vi "Apend Error Result to Case Element.vi"(8 "error in (no error)":errorcluster, 9 "Method Result":T1, 10 "Test Case Element in":refnum<k20>, 11 "XML Report In":refnum<class "XML Report.lvclass">) -> (0 "error out":errorcluster, 2 "Test Case Element out":refnum<k20>, 3 "XML Report Out":refnum<class "XML Report.lvclass">)   [LabVIEW 2020, in "XML Report.lvclass"]
uses:
  XML Report.lvclass
  <resource>/objmgr/DOMUserDefRef.rc
  <vilib>/xml/NI_XML.lvlib
  <vilib>/xml/Close Reference(Node).vi
  Result Types/Assertion Result/Public/TypeDefs/Status.ctl
  Result Types/Assertion Result/Assertion Result.lvlib
  Result Types/Assertion Result/Public/TypeDefs/Assertion Type.ctl
  Result Types/Assertion Result/Assertion Result.ctl
  Result Types/Method Result/Method Result.ctl
  Result Types/Method Result/Method Result.lvlib
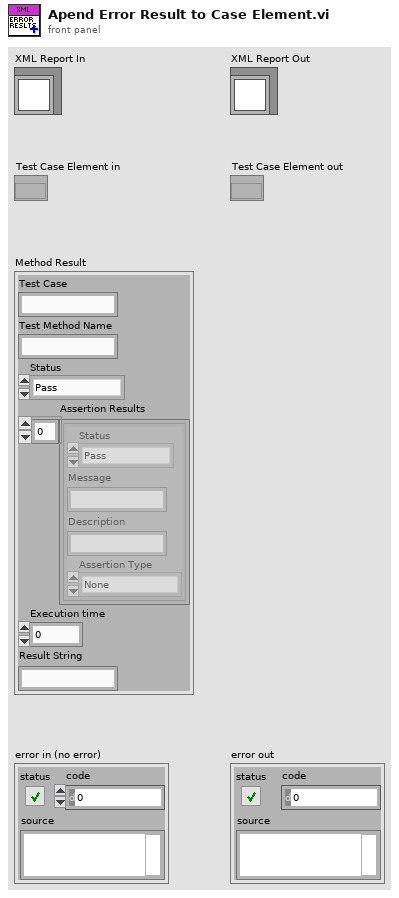
[diagram p1: front panel]
types:
  T1 = typedef "Method Result.lvlib/Method Result.ctl" = cluster{"Test Case":string, "Test Method Name":string, "Status":T2, "Assertion Results":T3[], "Execution time":dbl, "Result String":string}
  T2 = typedef "Assertion Result.lvlib/Status.ctl" = enum16{"Pass", "Fail", "Error", "Skipped", "Setup Error", "Broken", "Teardown Error"}
  T3 = typedef "Assertion Result.lvlib/Assertion Result.ctl" = cluster{"Status":T2, "Message":string, "Description":string, "Assertion Type":T4}
  T4 = typedef "Assertion Result.lvlib/Assertion Type.ctl" = enum16{"None", "Pass", "Fail", "Skip", "Pass if Equal", "Fail if Equal", "Pass if Error", "Fail if Error", "Pass if", "Fail if"}
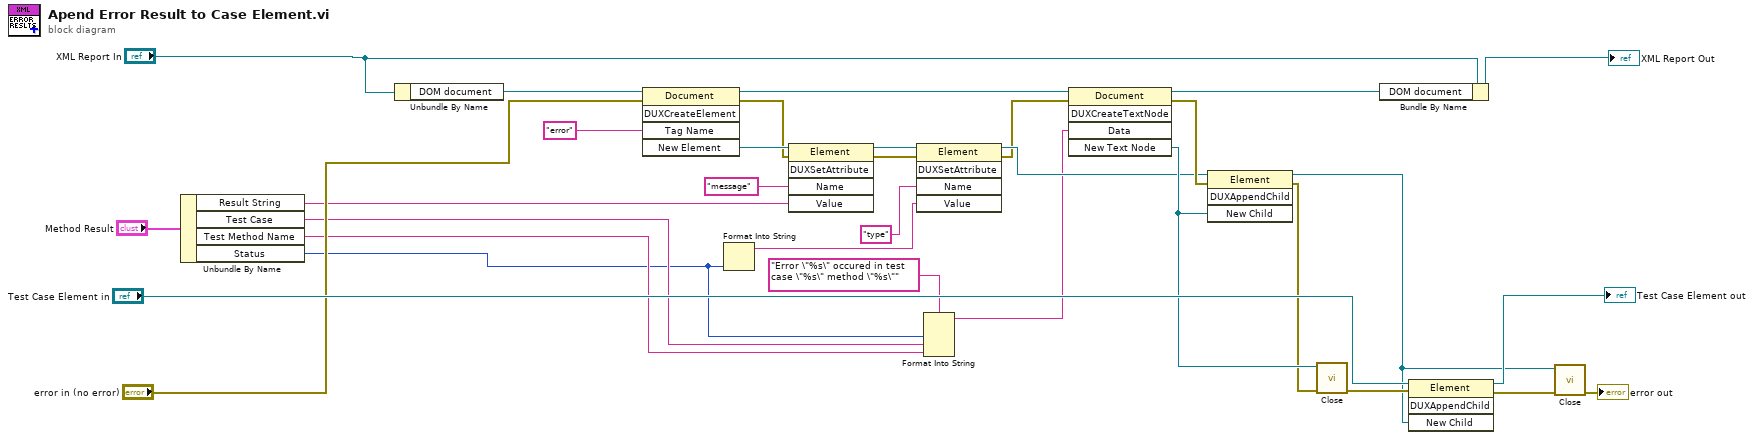
[diagram p0: block diagram]
diagram:
  n1 = Unbundle By Name("Method Result") -> ("Result String"=w5:string, "Test Case"=w3:string, "Test Method Name"=w2:string, "Status"=w1:T2)
  n2 = Unbundle By Name("XML Report In") -> ("DOM document"=w27:refnum<k20>)
  n3 = invoke class="Document" method="DUXCreateElement"(reference=w27, error in="error in (no error)", "Tag Name"="error") -> (reference out=w20:refnum<k20>, error out=w24:errorcluster, "New Element"=w25:refnum<k20>)  [unwired: 2 in, 2 out]
  n4 = Format Into String(w1) -> (resulting string=w9:string)  [unwired: 3 in, 1 out]
  n5 = invoke class="Element" method="DUXSetAttribute"(reference=w25, error in=w24, "Name"="message", "Value"=w5) -> (reference out=w13:refnum<k20>, error out=w11:errorcluster)  [unwired: 1 in, 3 out]
  n6 = invoke class="Element" method="DUXSetAttribute"(reference=w13, error in=w11, "Name"="type", "Value"=w9) -> (reference out=w12:refnum<k20>, error out=w10:errorcluster)  [unwired: 1 in, 3 out]
  n7 = Format Into String(format string="Error \"%s\" occured in test case \"%s\" method \"%s\"", w1, w3, w2) -> (resulting string=w7:string)  [unwired: 2 in, 1 out]
  n8 = invoke class="Document" method="DUXCreateTextNode"(reference=w20, error in=w10, "Data"=w7) -> (reference out=w19:refnum<k20>, error out=w21:errorcluster, "New Text Node"=w18:refnum<k20>)  [unwired: 2 in, 2 out]
  n9 = invoke class="Element" method="DUXAppendChild"(reference=w12, error in=w21, "New Child"=w18) -> (reference out=w15:refnum<k20>, error out=w17:errorcluster)  [unwired: 1 in, 2 out]
  n10 = call-poly <vilib>:"Close.vi"("error in (no error)"=w17, "node"=w18) -> ("error out"=w16:errorcluster)  [unwired: 7 in]
  n11 = Bundle By Name(cluster="XML Report In", "DOM document"=w19) -> (→"XML Report Out":refnum<class "XML Report.lvclass">)
  n12 = invoke class="Element" method="DUXAppendChild"(reference="Test Case Element in", error in=w16, "New Child"=w15) -> (reference out=→"Test Case Element out":refnum<k20>, error out=w22:errorcluster)  [unwired: 1 in, 2 out]
  n13 = call-poly <vilib>:"Close.vi"("error in (no error)"=w22, "node"=w15) -> ("error out"=→"error out":errorcluster)  [unwired: 7 in]
